vi "iWorx Event Marker SubVI.vi"(7 "Reset count (f)":bool, 11 "waveform in":waveform(dbl)) -> (0 "Button Press Duration":dbl, 1 "Two Edge Separation (rising)":dbl, 2 "Button State":bool, 3 "0-1 Waveform out":waveform(dbl), 4 "Falling Edge Times":timestamp[](array[timestamp]), 5 "Button Count":u32, 6 "Rising Edge Times":timestamp[](array[timestamp]))   [LabVIEW 2012]
doc: "This subVI is designed to work with the iWorx Event Marker. It takes in a waveform from the sensor and records timestamps for each rising and falling edge."
uses:
  <vilib>/ptbypt/NI_PtbyPt.lvlib
panel:
  in  "# of Timestamps to store":i32=10
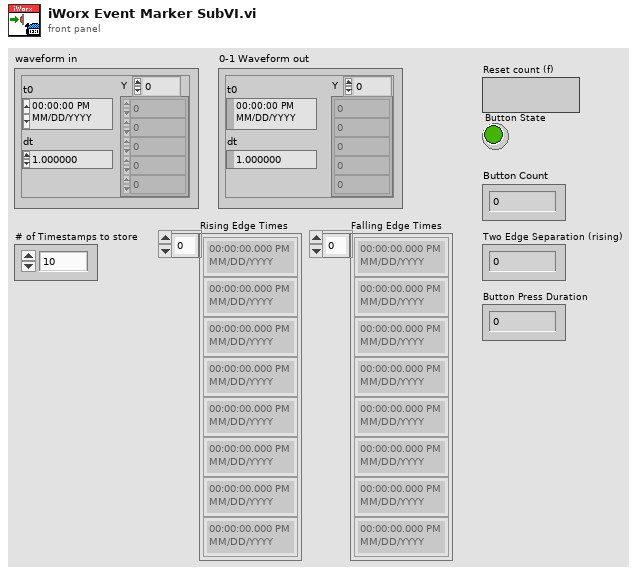
[diagram p1: front panel]
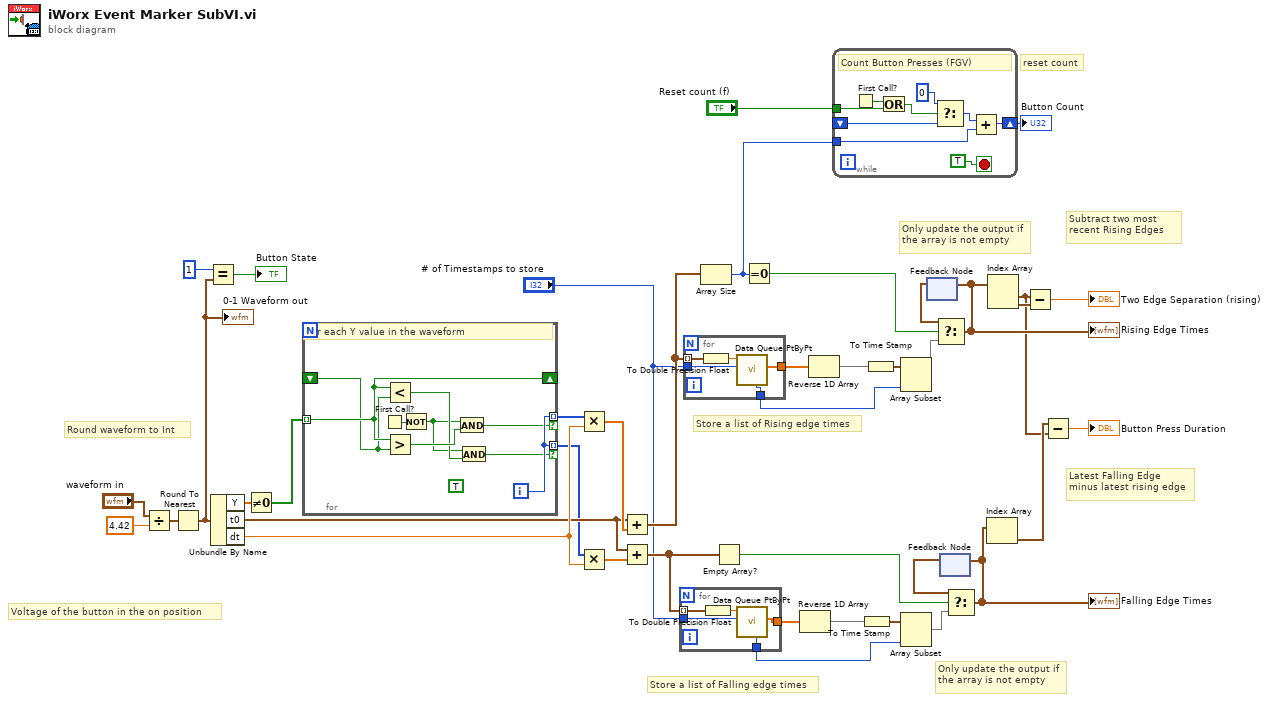
[diagram p0: block diagram]
diagram:
  # "reset count"
  # "Round waveform to Int"
  # "Latest Falling Edge minus latest rising edge"
  # "Subtract two most recent Rising Edges"
  # "Only update the output if the array is not empty"
  # "Only update the output if the array is not empty"
  # "Store a list of Rising edge times"
  # "Store a list of Falling edge times"
  # "Voltage of the button in the on position"
  n1 = Divide(x="waveform in", y=4.42) -> (x/y=w15:waveform(dbl))
  n2 = Round To Nearest(number=w15) -> (nearest integer value=w14:waveform(dbl))
  "0-1 Waveform out" <- w14
  n3 = Equal?(x=u8 1, y=w14) -> (x = y?=→"Button State":bool)
  n4 = Unbundle By Name(w14) -> ("Y"=w39:dbl[], "t0"=w33:timestamp, "dt"=w36:dbl)
  n5 = Not Equal To 0?(x=w39) -> (x != 0?=w38:bool[])
  n6 = for {
    tunnel: [w50] -> w32 mode=indexing if=w49
    tunnel: [w50] -> w37 mode=indexing if=w48
    tunnel: w38 -> [w47] mode=indexing
    shift-right: [w47] -> _
    shift-left: _ -> [w46]
    i -> [w50]
    (unwired) TRUE
    # "For each Y value in the waveform"
    n7 = First Call?() -> (First Call?: T/F=w42:bool)
    n8 = Less?(x=w47, y=w46) -> (x < y?=w44:bool)
    n9 = Greater?(x=w47, y=w46) -> (0:w45:bool)
    n10 = Not(x=w42) -> (.not. x?=w43:bool)
    n11 = And(x=w43, y=w45) -> (x .and. y?=w48:bool)
    n12 = And(x=w43, y=w44) -> (x .and. y?=w49:bool)
  }
  n13 = Multiply(x=w37, y=w36) -> (x*y=w35:dbl[])
  n14 = Multiply(x=w32, y=w36) -> (x*y=w34:dbl[])
  n15 = Add(x=w33, y=w35) -> (x+y=w28:timestamp[])
  n16 = Add(x=w33, y=w34) -> (x+y=w7:timestamp[])
  n17 = for {
    tunnel: w7 -> [w54] mode=indexing
    tunnel: "# of Timestamps to store" -> [w55]
    tunnel: [w52] -> w2
    tunnel: [w51] -> w9
    n18 = To Double Precision Float(number=w54) -> (double precision float=w53:dbl)
    n19 = call <vilib>:"Data Queue PtByPt.vi"("sample length"=w55, "input data point"=w53) -> ("Current Queue"=w52:dbl[], "current length"=w51:i32)  [unwired: 5 in, 3 out]
  }
  n20 = for {
    tunnel: w28 -> [w59] mode=indexing
    tunnel: "# of Timestamps to store" -> [w60]
    tunnel: [w57] -> w4
    tunnel: [w56] -> w11
    n21 = To Double Precision Float(number=w59) -> (double precision float=w58:dbl)
    n22 = call <vilib>:"Data Queue PtByPt.vi"("sample length"=w60, "input data point"=w58) -> ("Current Queue"=w57:dbl[], "current length"=w56:i32)  [unwired: 5 in, 3 out]
  }
  n23 = Array Size(array=w28) -> (size(s)=w27:i32)
  n24 = Empty Array?(array=w7) -> (empty?=w17:bool)
  n25 = Equal To 0?(x=w27) -> (x = 0?=w22:bool)
  n26 = Reverse 1D Array(array=w2) -> (reversed array=w1:dbl[])
  n27 = Reverse 1D Array(array=w4) -> (reversed array=w3:dbl[])
  n28 = while {
    shift-right: [w61] -> w26
    shift-left: _ -> [w63]
    tunnel: w27 -> [w65]
    tunnel: "Reset count (f)" -> [w64]
    stop <- TRUE stop-if-true
    # "Count Button Presses (FGV)"
    n29 = First Call?() -> (First Call?: T/F=w68:bool)
    n30 = Or(x=w68, y=w64) -> (x .or. y?=w66:bool)
    n31 = Select(t=u32 0, s=w66, f=w63) -> (s? t:f=w62:u32)
    n32 = Add(x=w62, y=w65) -> (x+y=w61:u32)
  }
  "Button Count" <- w26
  n33 = To Time Stamp(1:w1) -> (0:w8:timestamp[])
  n34 = To Time Stamp(1:w3) -> (0:w12:timestamp[])
  n35 = Array Subset(array=w12, length=w11) -> (w10:timestamp[])  [unwired: 1 in]
  n36 = Array Subset(array=w8, length=w9) -> (w5:timestamp[])  [unwired: 1 in]
  n37 = feedback #1() -> (w31:timestamp[])  [unwired: 1 in]
  n38 = Select(t=w31, s=w22, f=w10) -> (s? t:f=w30:timestamp[])
  "Rising Edge Times" <- w30
  n39 = feedback-in #1(w30) -> ()
  n40 = feedback #2() -> (w29:timestamp[])  [unwired: 1 in]
  n41 = Select(t=w29, s=w17, f=w5) -> (s? t:f=w21:timestamp[])
  "Falling Edge Times" <- w21
  n42 = feedback-in #2(w21) -> ()
  n43 = Index Array(array=w21) -> (element=w19:timestamp)  [unwired: 1 in]
  n44 = Index Array(array=w30) -> (element #1=w18:timestamp, element #2=w40:timestamp)  [unwired: 2 in]
  n45 = Subtract(x=w18, y=w40) -> (x-y=→"Two Edge Separation (rising)":dbl)
  n46 = Subtract(x=w19, y=w18) -> (x-y=→"Button Press Duration":dbl)
